vi "Remove Rows.vi"(4 "Rows":i32[](array[numeric]), 6 "Mode":enum16{"Selected Rows", "Input Rows"}(ring), 8 "error in (no error)":errorcluster, 10 "DataGridView in":refnum<class "DataGridView.lvclass">, 11 "Numeric Control":i32) -> (0 "error out":errorcluster)   [LabVIEW 2013, in "DataGrid.lvlib" / "DataGridView.lvclass"]
doc: "This VI allows you to remove rows from the data table. The mode input chooses if you are removing specific rows or selected rows."
uses:
  DataGridView.lvclass
  DataGridView.lvclass/DataGridView.ctl
  System.Windows.Forms
  Properties/Read DataGridView.vi
  Properties/Read SelectionMode.vi
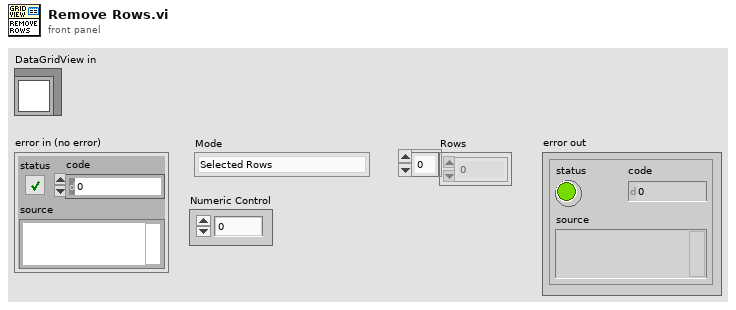
[diagram p1: front panel]
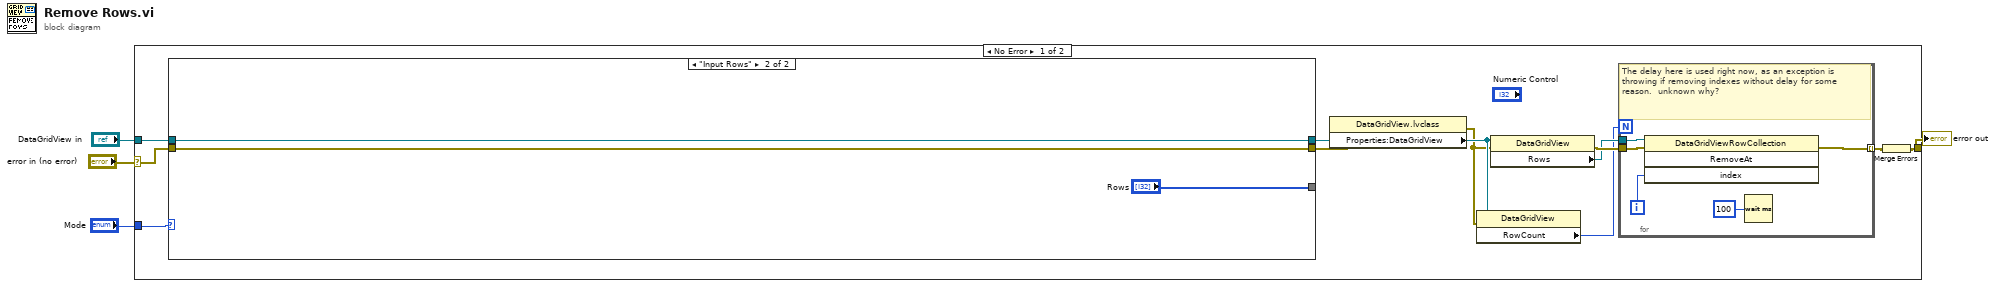
[diagram p0: block diagram]
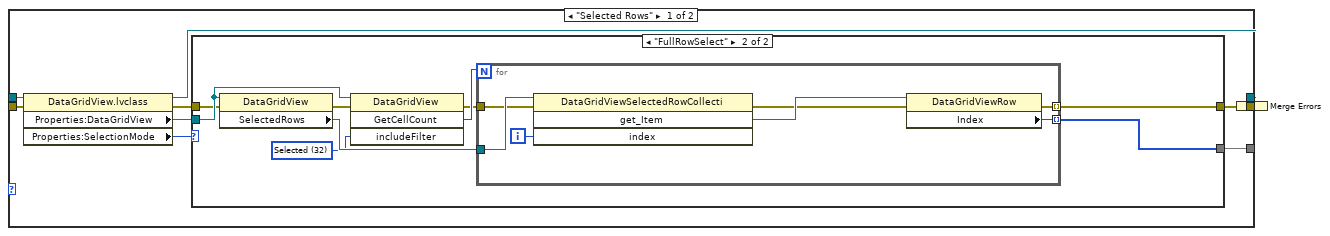
[diagram p2: hidden frame]
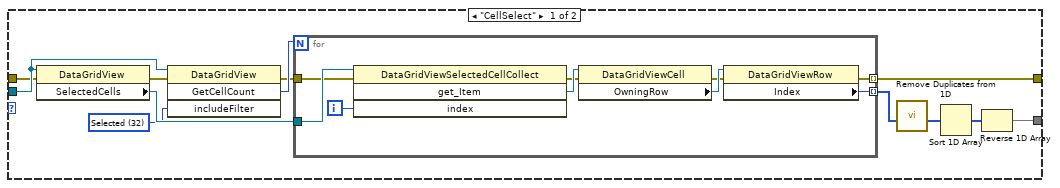
[diagram p3: hidden frame]
diagram:
  n1 = case shown="No Error" "error in (no error)" {
    selector: "error in (no error)" -> [w12 w71]
    tunnel: "DataGridView in" -> [w16 _]
    tunnel: "Mode" -> [w13 _]
    tunnel: [w10 w71] -> w1
    frame No Error {
      n2 = case shown="\"Input Rows\"" w13 {
        tunnel: w16 -> [w25 w63]
        tunnel: [w18 w64] -> w11
        tunnel: [w23 "Rows"] -> _
        tunnel: w12 -> [w19 w64]
        tunnel: [w17 w63] -> w9
        frame "Selected Rows" {
          n3 = property class="DataGridView.lvclass"(reference=w25, error in=w19) -> (reference out=w17:refnum<class "DataGridView.lvclass">, error out=w21:errorcluster, "Properties:DataGridView"=w22:refnum<k24>, "Properties:SelectionMode"=w20:enum16{"CellSelect", "FullRowSelect"})
          n4 = case shown="\"FullRowSelect\"" w20 {
            tunnel: [w36 w54] -> w24
            tunnel: [w28 w53] -> w23
            tunnel: w22 -> [w35 w52]
            tunnel: w21 -> [w30 w47]
            frame "CellSelect" {
              w34 = 32 items=["None"=0, "Displayed"=1, "Frozen"=2, "ReadOnly"=4, "Resizable"=8, "ResizableSet"=16, "Selected"=32, "Visible"=64] ("includeFilter")
              n5 = property class="DataGridView"(reference=w35, error in=w30) -> (error out=w32:errorcluster, "SelectedCells"=w37:refnum<k24>)  [unwired: 1 out]
              n6 = invoke class="DataGridView" method="GetCellCount"(reference=w35, error in=w32, "includeFilter"=w34) -> (error out=w31:errorcluster, "GetCellCount"=w33:i32)  [unwired: 1 in, 2 out]
              n7 = for {
                N: w33 -> [_]
                tunnel: w37 -> [w43]
                tunnel: [w41] -> w27 mode=indexing
                tunnel: [w39] -> w36 mode=indexing
                tunnel: w31 -> [w38]
                i -> [w45]
                n8 = invoke class="DataGridViewSelectedCellCollect" method="get_Item"(reference=w43, error in=w38, "index"=w45) -> (error out=w44:errorcluster, "get_Item"=w46:refnum<k24>)  [unwired: 1 in, 2 out]
                n9 = property class="DataGridViewCell"(reference=w46, error in=w44) -> (error out=w40:errorcluster, "OwningRow"=w42:refnum<k24>)  [unwired: 1 out]
                n10 = property class="DataGridViewRow"(reference=w42, error in=w40) -> (error out=w39:errorcluster, "Index"=w41:i32)  [unwired: 1 out]
              }
              n11 = call "Remove Duplicates from 1D.vi"("Input Array"=w27) -> ("No Duplicates Array"=w26:i32[])  [unwired: 10 in]
              n12 = Sort 1D Array(array=w26) -> (sorted array=w29:i32[])
              n13 = Reverse 1D Array(array=w29) -> (reversed array=w28:i32[])
            }
            frame "FullRowSelect" {
              w51 = 32 items=["None"=0, "Displayed"=1, "Frozen"=2, "ReadOnly"=4, "Resizable"=8, "ResizableSet"=16, "Selected"=32, "Visible"=64] ("includeFilter")
              n14 = property class="DataGridView"(reference=w52, error in=w47) -> (error out=w49:errorcluster, "SelectedRows"=w55:refnum<k24>)  [unwired: 1 out]
              n15 = invoke class="DataGridView" method="GetCellCount"(reference=w52, error in=w49, "includeFilter"=w51) -> (error out=w48:errorcluster, "GetCellCount"=w50:i32)  [unwired: 1 in, 2 out]
              n16 = for {
                N: w50 -> [_]
                tunnel: w55 -> [w61]
                tunnel: [w60] -> w53 mode=indexing
                tunnel: [w59] -> w54 mode=indexing
                tunnel: w48 -> [w58]
                i -> [w62]
                n17 = invoke class="DataGridViewSelectedRowCollecti" method="get_Item"(reference=w61, error in=w58, "index"=w62) -> (error out=w56:errorcluster, "get_Item"=w57:refnum<k24>)  [unwired: 1 in, 2 out]
                n18 = property class="DataGridViewRow"(reference=w57, error in=w56) -> (error out=w59:errorcluster, "Index"=w60:i32)  [unwired: 1 out]
              }
            }
          }
          n19 = Merge Errors(w24) -> (w18:errorcluster)
        }
        frame "Input Rows" {
        }
      }
      n20 = property class="DataGridView.lvclass"(reference=w9, error in=w11) -> (error out=w6:errorcluster, "Properties:DataGridView"=w7:refnum<k24>)  [unwired: 1 out]
      n21 = property class="DataGridView"(reference=w7, error in=w6) -> ("RowCount"=w5:i32)  [unwired: 2 out]
      n22 = property class="DataGridView"(reference=w7, error in=w6) -> (error out=w15:errorcluster, "Rows"=w8:refnum<k24>)  [unwired: 1 out]
      n23 = for {
        N: w5 -> [_]
        tunnel: w15 -> [w70]
        tunnel: [w66] -> w14 mode=indexing
        tunnel: w8 -> [w68]
        i -> [w67]
        # "The delay here is used right now, as an exception is throwing if removing indexes without delay for some reason.  unknown why?"
        n24 = invoke class="DataGridViewRowCollection" method="RemoveAt"(reference=w68, error in=w70, "index"=w67) -> (error out=w66:errorcluster)  [unwired: 1 in, 3 out]
        n25 = Wait (ms)(milliseconds to wait=u32 100) -> ()  [unwired: 1 out]
      }
      n26 = Merge Errors(w14) -> (w10:errorcluster)
    }
    frame Error {
    }
  }
  "error out" <- w1
